vi "EnableOutput.vi"(8 "error in (no error)":errorcluster, 11 "Sync Box in":refnum<class "Sync Box.lvclass">) -> (0 "error out":errorcluster, 3 "Sync Box out":refnum<class "Sync Box.lvclass">)   [LabVIEW 2018, in "Sync Box.lvclass"]
uses:
  Sync Box.lvclass
  Sync Box.lvclass/Sync Box.ctl
  Trigger/Trigger.lvclass/Trigger.ctl
  Trigger/Trigger.lvclass
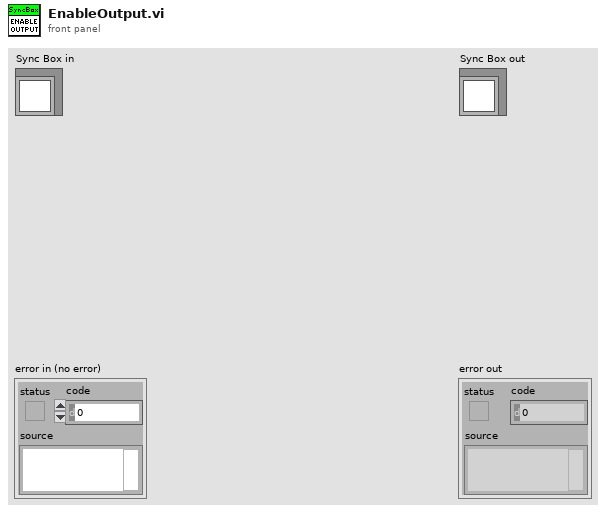
[diagram p1: front panel]
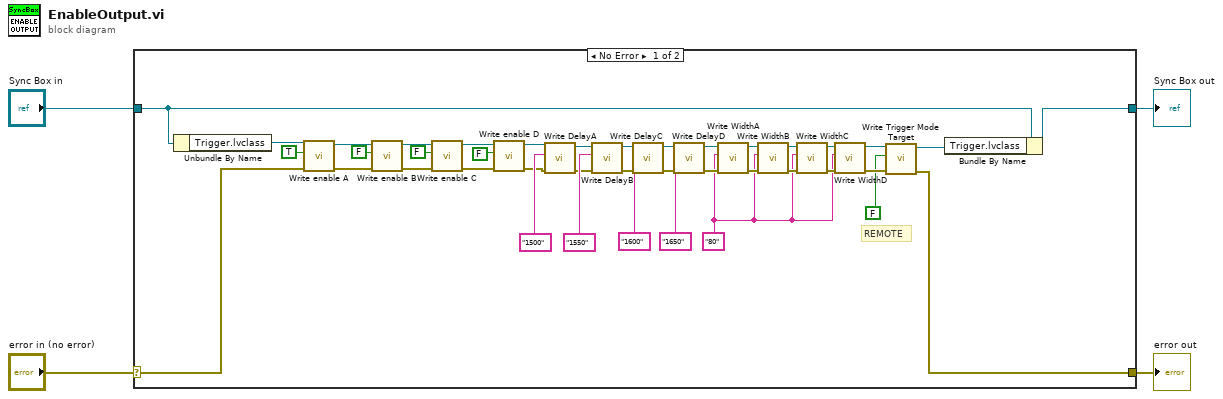
[diagram p0: block diagram]
diagram:
  n1 = case shown="No Error" "error in (no error)" {
    selector: "error in (no error)" -> [w35 w46]
    tunnel: [w6 w46] -> w3
    tunnel: [w43 w45] -> w1
    tunnel: "Sync Box in" -> [w44 w45]
    frame No Error {
      w10 = "80" ("DelayA")
      # "REMOTE"
      n2 = Unbundle By Name(w44) -> ("Trigger.lvclass"=w42:refnum<class "Trigger.lvclass">)
      n3 = call "Write enable A.vi"("error in (no error)"=w35, "enable A"=TRUE, "Trigger in"=w42) -> ("error out"=w38:errorcluster, "Trigger out"=w41:refnum<class "Trigger.lvclass">)  [unwired: 7 in]
      n4 = call "Write enable B.vi"("error in (no error)"=w38, "enable B"=FALSE, "Trigger in"=w41) -> ("error out"=w37:errorcluster, "Trigger out"=w40:refnum<class "Trigger.lvclass">)  [unwired: 7 in]
      n5 = call "Write enable C.vi"("error in (no error)"=w37, "enable C"=FALSE, "Trigger in"=w40) -> ("error out"=w36:errorcluster, "Trigger out"=w39:refnum<class "Trigger.lvclass">)  [unwired: 7 in]
      n6 = call "Write enable D.vi"("error in (no error)"=w36, "enable D"=FALSE, "Trigger in"=w39) -> ("error out"=w19:errorcluster, "Trigger out"=w30:refnum<class "Trigger.lvclass">)  [unwired: 7 in]
      n7 = call-dynamic "Write DelayA.vi"("error in (no error)"=w19, "DelayA"="1500", "Trigger in"=w30) -> ("error out"=w18:errorcluster, "Trigger out"=w29:refnum<class "Trigger.lvclass">)  [unwired: 7 in]
      n8 = call-dynamic "Write DelayB.vi"("error in (no error)"=w18, "DelayB"="1550" ("DelayA"), "Trigger in"=w29) -> ("error out"=w17:errorcluster, "Trigger out"=w28:refnum<class "Trigger.lvclass">)  [unwired: 7 in]
      n9 = call-dynamic "Write DelayC.vi"("error in (no error)"=w17, "DelayC"="1600" ("DelayA"), "Trigger in"=w28) -> ("error out"=w16:errorcluster, "Trigger out"=w27:refnum<class "Trigger.lvclass">)  [unwired: 7 in]
      n10 = call-dynamic "Write DelayD.vi"("error in (no error)"=w16, "DelayD"="1650" ("DelayA"), "Trigger in"=w27) -> ("error out"=w15:errorcluster, "Trigger out"=w26:refnum<class "Trigger.lvclass">)  [unwired: 7 in]
      n11 = call-dynamic "Write WidthA.vi"("error in (no error)"=w15, "WidthA"=w10, "Trigger in"=w26) -> ("error out"=w14:errorcluster, "Trigger out"=w25:refnum<class "Trigger.lvclass">)  [unwired: 7 in]
      n12 = call-dynamic "Write WidthB.vi"("error in (no error)"=w14, "WidthB"=w10, "Trigger in"=w25) -> ("error out"=w13:errorcluster, "Trigger out"=w24:refnum<class "Trigger.lvclass">)  [unwired: 7 in]
      n13 = call-dynamic "Write WidthC.vi"("error in (no error)"=w13, "WidthC"=w10, "Trigger in"=w24) -> ("error out"=w12:errorcluster, "Trigger out"=w11:refnum<class "Trigger.lvclass">)  [unwired: 7 in]
      n14 = call-dynamic "Write WidthD.vi"("error in (no error)"=w12, "WidthD"=w10, "Trigger in"=w11) -> ("error out"=w7:errorcluster, "Trigger out"=w9:refnum<class "Trigger.lvclass">)  [unwired: 7 in]
      n15 = call-dynamic "Write Trigger Mode Target.vi"("error in (no error)"=w7, "Trigger Mode Target"=FALSE, "Trigger in"=w9) -> ("error out"=w6:errorcluster, "Trigger out"=w8:refnum<class "Trigger.lvclass">)  [unwired: 7 in]
      n16 = Bundle By Name(cluster=w44, "Trigger.lvclass"=w8) -> (w43:refnum<class "Sync Box.lvclass">)
    }
    frame Error {
    }
  }
  "error out" <- w3
  "Sync Box out" <- w1
